vi "WAV_Convert.vi"(10 "data":waveform(dbl)[](array[waveform]), 11 "bit depth":u16=32) -> (0 "Data":waveform(sgl)[](graph), 2 "Data":sgl[][](array[numeric]), 3 "format":T1)   [LabVIEW 2022 SP3]
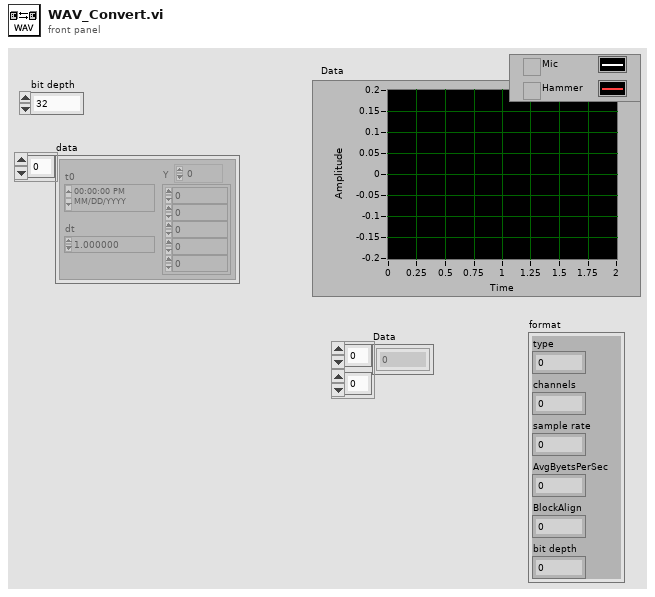
[diagram p1: front panel]
types:
  T1 = cluster{"type":u16, "channels":u16, "sample rate":u32, "AvgByetsPerSec":u32, "BlockAlign":u16, "bit depth":u16}
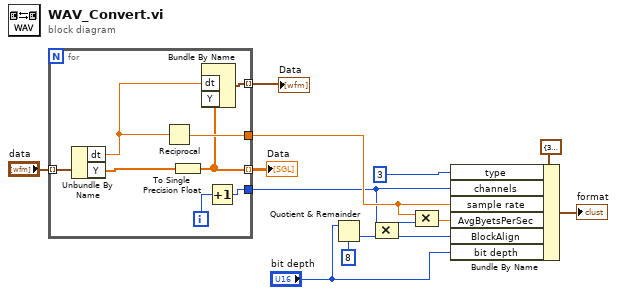
[diagram p0: block diagram]
diagram:
  n1 = for {
    tunnel: "data" -> [w21] mode=indexing
    tunnel: [w15] -> w11 mode=indexing
    tunnel: [w19] -> w5
    tunnel: [w18] -> w13
    tunnel: [w14] -> w1 mode=indexing
    i -> [w20]
    n2 = Unbundle By Name(w21) -> ("dt"=w16:dbl, "Y"=w17:dbl[])
    n3 = Reciprocal(x=w16) -> (1/x=w18:dbl)
    n4 = To Single Precision Float(number=w17) -> (single precision float=w15:sgl[])
    n5 = Bundle By Name("dt"=w16, "Y"=w15) -> (w14:waveform(sgl))  [unwired: 1 in]
    n6 = Increment(x=w20) -> (x+1=w19:i32)
  }
  "Data" <- w1
  "Data" <- w11
  n7 = Quotient & Remainder(x="bit depth", y=u16 8 ("bit depth")) -> (floor(x/y)=w3:u16)  [unwired: 1 out]
  n8 = Compound Arithmetic op=MULTIPLY(w5, w3) -> (w6:i32)
  n9 = Compound Arithmetic op=MULTIPLY(w13, w6) -> (w7:dbl)
  n10 = Bundle By Name(cluster=T1 {"type"=3, "channels"=1, "sample rate"=44100, "AvgByetsPerSec"=176400, "BlockAlign"=4, "bit depth"=32} ("format"), "type"=u16 3, "channels"=w5, "sample rate"=w13, "AvgByetsPerSec"=w7, "BlockAlign"=w6, "bit depth"="bit depth") -> (→"format":T1)
